vi "Miniquads.Initialize.vi"(0 "i ref in":refnum<vi>, 3 "ms timeout (10000)":i32=10000, 5 "error in (no error)":errorcluster) -> (14 "i ref out":refnum<vi>, 15 "DeviceID":string, 17 "timed out":bool, 19 "error out":errorcluster)   [LabVIEW 2014, in "Miniquads.lvlib"]
doc: "This vi initializes the used objects and reads the device id."
uses:
  Miniquads.lvlib
  CSCore/BaseProcess/BaseProcess.lvlib
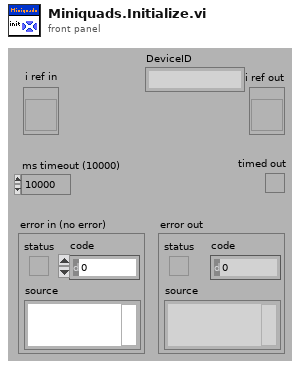
[diagram p1: front panel]
types:
  T1 = typedef "Miniquads.lvlib/Miniquads.i attribute.ctl" = cluster{"ObjectsInitialized":bool, "ObjectsLoaded":string[], "nomValues":T2, "actValues":T2}
  T2 = typedef "Miniquads.lvlib/Miniquads.voltages.ctl" = cluster{"FocusVoltage":dbl, "HorizontalVoltage":dbl, "VerticalVoltage":dbl, "serviceIDs":cluster{"FocusVoltageID":i32, "HorizontalVoltageID":i32, "VerticalVoltageID":i32}}
  T3 = typedef "BaseProcess.lvlib/BaseProcess.i attribute.ctl" = cluster{"EventStatus":string, "EventError":i32, "PresetEvtWatchD":i32, "PresetPdcWatchD":i32, "EventTimeout":i32, "PeriodicInterval":i32, "Interface":string[], "Address":string[], "Special":string[], "PeriodicError":i32, "PeriodicStatus":string, "SuperProc":string, "Descriptors":T4[], "CaseRef":refnum<vi>, "PdcRef":refnum<vi>, "Thread Ref":refnum<vi>, "eventErrorID":i32, "eventStatusID":i32, "periodicErrorID":i32, "periodicStatusID":i32, "pdcCtrID":i32}
  T4 = typedef "BaseProcess.lvlib/BaseProcess.descriptor definition.ctl" = cluster{"selector":string, "descriptor":T5}
  T5 = typedef "BaseProcess.lvlib/BaseProcess.descriptor string definition.ctl" = string
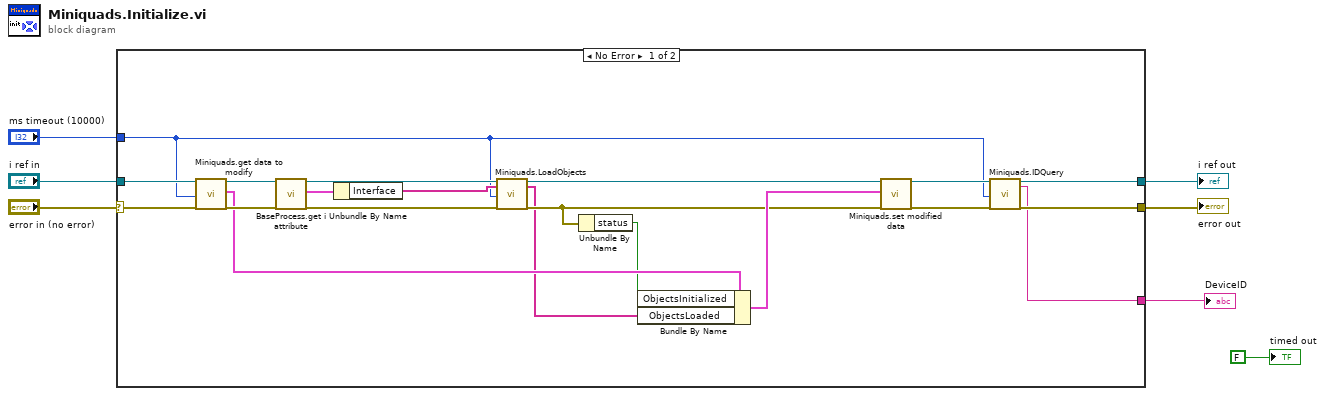
[diagram p0: block diagram]
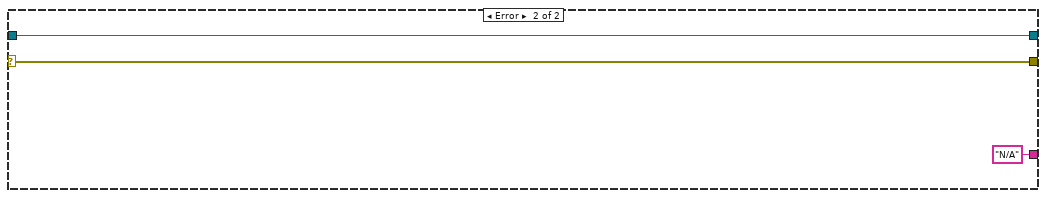
[diagram p2: hidden frame]
diagram:
  n1 = case shown="No Error" "error in (no error)" {
    selector: "error in (no error)" -> [w26 w29]
    tunnel: "i ref in" -> [w27 w30]
    tunnel: [w11 w30] -> w6
    tunnel: [w10 w29] -> w4
    tunnel: "ms timeout (10000)" -> [w8 _]
    tunnel: [w9 "N/A"] -> w1
    frame No Error {
      n2 = call "Miniquads.get data to modify.vi"("i ref in"=w27, "ms timeout (10000)"=w8, "error in (no error)"=w26) -> ("i ref out"=w25:refnum<vi>, "i attribute"=w20:T1, "error out"=w24:errorcluster)  [unwired: 13 in, 1 out]
      n3 = call "BaseProcess.get i attribute.vi"("i ref in"=w25, "error in (no error)"=w24) -> ("i ref out"=w22:refnum<vi>, "i attribute"=w23:T3, "error out"=w21:errorcluster)  [unwired: 15 in]
      n4 = Unbundle By Name(w23) -> ("Interface"=w14:string[])
      n5 = call "Miniquads.LoadObjects.vi"("i ref in"=w22, "Objects"=w14, "ms timeout (10000)"=w8, "error in (no error)"=w21) -> ("i ref out"=w19:refnum<vi>, "ObjectsLoaded"=w15:string[], "error out"=w17:errorcluster)  [unwired: 12 in, 1 out]
      n6 = Unbundle By Name(w17) -> ("status"=w16:bool)
      n7 = Bundle By Name(cluster=w20, "ObjectsInitialized"=w16, "ObjectsLoaded"=w15) -> (w18:T1)
      n8 = call "Miniquads.set modified data.vi"("i ref in"=w19, "i attribute"=w18, "error in (no error)"=w17) -> ("i ref out"=w13:refnum<vi>, "error out"=w12:errorcluster)  [unwired: 15 in]
      n9 = call "Miniquads.IDQuery.vi"("i ref in"=w13, "ms timeout (10000)"=w8, "error in (no error)"=w12) -> ("i ref out"=w11:refnum<vi>, "DeviceID"=w9:string, "error out"=w10:errorcluster)  [unwired: 13 in, 1 out]
    }
    frame Error {
    }
  }
  "error out" <- w4
  "i ref out" <- w6
  "DeviceID" <- w1
  "timed out" <- FALSE ("timed out")
